vi "GitDetailedLog.vi"(6 "skip":i32 min=0 step=1, 8 "error in (no error)":errorcluster, 9 "Directory":path=path "", 10 "Number":i32=1 min=1 step=1, 11 "Git exec":string="git") -> (0 "error out":errorcluster, 1 "Directory out":path, 2 "Detail Array":string[][](array[string]), 3 "Git exec out":string="git")   [LabVIEW 2013]
uses:
  <vilib>/Utility/error.llb/whitespace.ctl
  GitCommitCluster/CommitCluster.ctl
  GitCmd.vi
  <vilib>/dlg_ctls.llb/Space Constant.vi
  GitUtils/PathtoDirPath.vi
  <vilib>/Platform/system.llb/System Exec.vi
  <vilib>/Utility/error.llb/Error Cluster From Error Code.vi
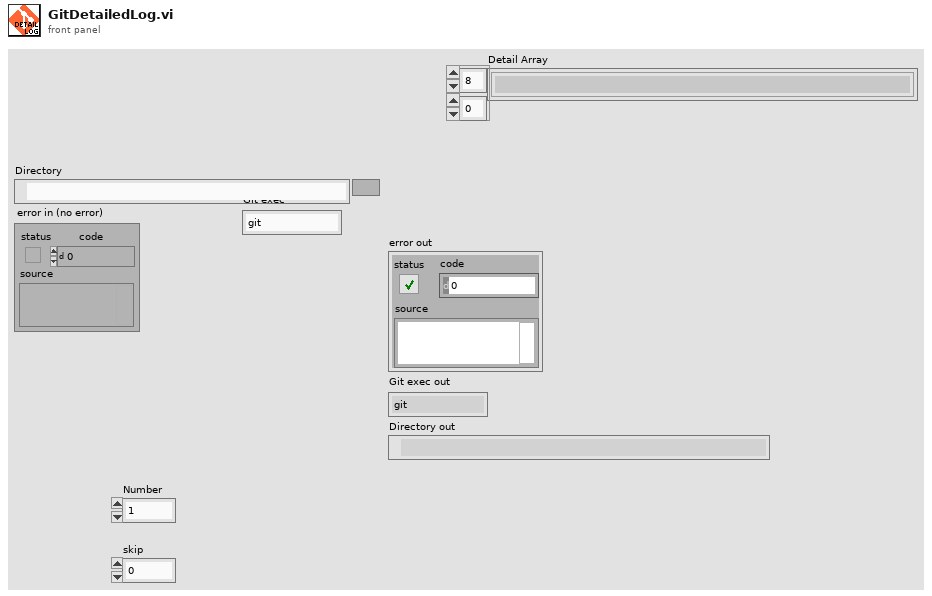
[diagram p1: front panel]
types:
  T1 = typedef "whitespace.ctl" = u16
  T2 = typedef "CommitCluster.ctl" = cluster{"Hash":string, "Date":string, "Name":string}
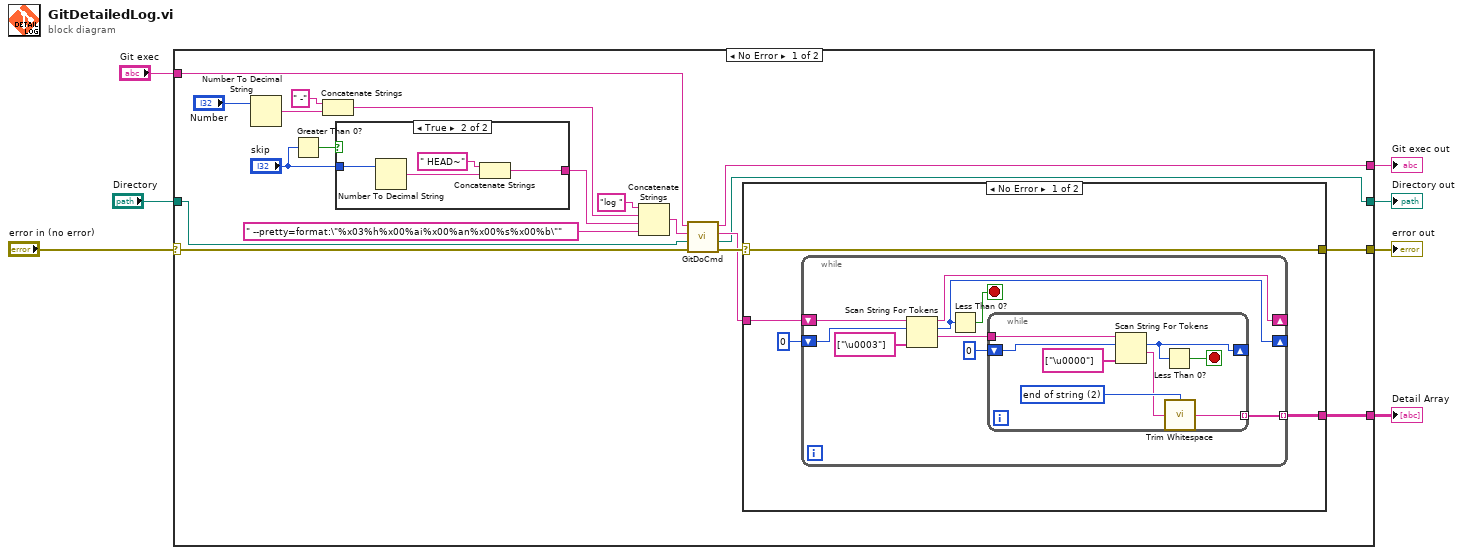
[diagram p0: block diagram]
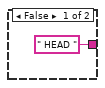
[diagram p2: hidden frame]
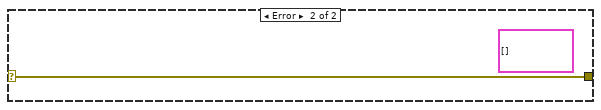
[diagram p3: hidden frame]
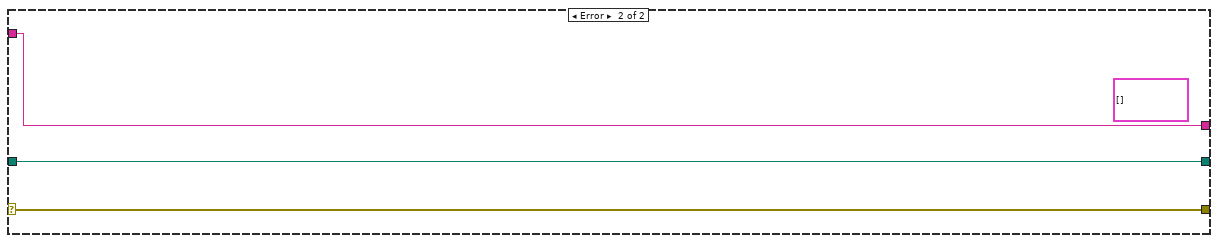
[diagram p4: hidden frame]
diagram:
  n1 = case shown="No Error" "error in (no error)" {
    selector: "error in (no error)" -> [w16 w56]
    tunnel: "Git exec" -> [w13 w55]
    tunnel: "Directory" -> [w9 w54]
    tunnel: [w17 w56] -> w5
    tunnel: [w12 w55] -> w3
    tunnel: [w10 w54] -> w2
    tunnel: [w8 _] -> w1
    frame No Error {
      n2 = Number To Decimal String(number="Number") -> (decimal integer string=w24:string)  [unwired: 1 in]
      n3 = Greater Than 0?(x="skip") -> (x > 0?=w21:bool)
      n4 = Concatenate Strings(" -" ("string"), w24) -> (w22:string)
      n5 = case shown="True" w21 {
        tunnel: "skip" -> [_ w31]
        tunnel: [" HEAD " w28] -> w19
        frame False {
        }
        frame True {
          n6 = Number To Decimal String(number=w31) -> (decimal integer string=w30:string)  [unwired: 1 in]
          n7 = Concatenate Strings(" HEAD~" ("string"), w30) -> (w28:string)
        }
      }
      n8 = Concatenate Strings("log " ("string"), w22, w19, " --pretty=format:\"%x03%h%x00%ai%x00%an%x00%s%x00%b\"" ("string")) -> (w14:string)
      n9 = call "GitDoCmd.vi"("error in (no error)"=w16, "Working Path"=w9, "Git command"=w14, "Git exec"=w13) -> ("error out"=w15:errorcluster, "Working Path out"=w10:path, "Returned stdout"=w11:string, "Git exec out"=w12:string)  [unwired: 3 in]
      n10 = case shown="No Error" w15 {
        selector: w15 -> [w35 w53]
        tunnel: w11 -> [w34 _]
        tunnel: [w35 w53] -> w17
        tunnel: [w33 _] -> w8
        frame No Error {
          n11 = while {
            shift-right: [w42] -> _
            shift-left: w34 -> [w44]
            tunnel: [w37] -> w33 mode=indexing
            shift-right: [w39] -> _
            shift-left: 0 ("offset past token") -> [w41]
            stop <- w40 stop-if-true
            n12 = Scan String For Tokens(6:string[] ["\u0003"] ("delimiters (\\s,\\t,\\r,\\n)"), 8:w41, 9:w44) -> (1:w38:string, 2:w39:i32, 3:w42:string)  [unwired: 3 in, 1 out]
            n13 = Less Than 0?(x=w39) -> (x < 0?=w40:bool)
            n14 = while {
              tunnel: w38 -> [w50]
              tunnel: [w45] -> w37 mode=indexing
              shift-right: [w49] -> _
              shift-left: 0 ("offset past token") -> [w48]
              stop <- w51 stop-if-true
              w47 = T1 2 items=["both", "start of string", "end of string"] ("location (both)")
              n15 = Scan String For Tokens(6:string[] ["\u0000"] ("delimiters (\\s,\\t,\\r,\\n)"), 8:w48, 9:w50) -> (1:w46:string, 2:w49:i32)  [unwired: 3 in, 2 out]
              n16 = Less Than 0?(x=w49) -> (x < 0?=w51:bool)
              n17 = call <vilib>:"Trim Whitespace.vi"("string"=w46, "location (both)"=w47) -> ("trimmed string"=w45:string)
            }
          }
        }
        frame Error {
          (unwired) T2[] [] ("Array")
        }
      }
    }
    frame Error {
      (unwired) T2[] [] ("Array")
    }
  }
  "error out" <- w5
  "Git exec out" <- w3
  "Directory out" <- w2
  "Detail Array" <- w1
